vi "Get Tester Info.vi"(0 "TSM Context In":T1, 5 "Tester Type":string="RFPM", 11 "error in":errorcluster) -> (4 "TSM Context Out":T1, 6 "Resource Descriptors Exist?":bool, 8 "Resource Descriptors":string[](array[string]), 10 "Instrument Models":string[](array[string]), 15 "error out":errorcluster)   [LabVIEW 2023, in "RFCalAndFixtureCharact.Common.lvlib"]
uses:
  RFCalAndFixtureCharact.Common.lvlib
  <vilib>/NI_TestStand_SemiconductorModule/NI_TestStand_Semiconductor_Module.lvlibp/PinMap/General/SemiconductorModuleContext.ctl
  Global Data Id Prefix.vi
  <vilib>/NI_TestStand_SemiconductorModule/NI_TestStand_Semiconductor_Module.lvlibp
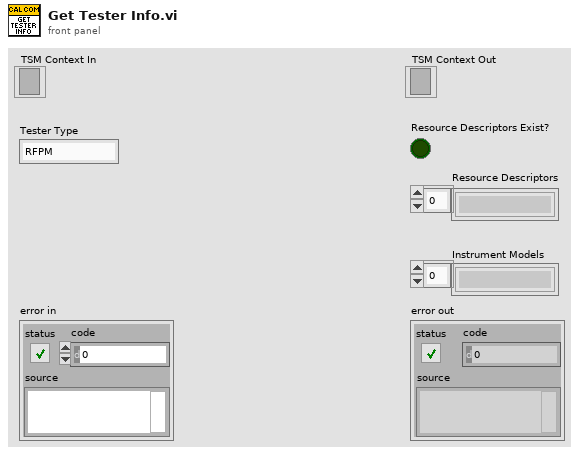
[diagram p1: front panel]
types:
  T1 = typedef "NI_TestStand_Semiconductor_Module.lvlibp/SemiconductorModuleContext.ctl" = refnum<k7>
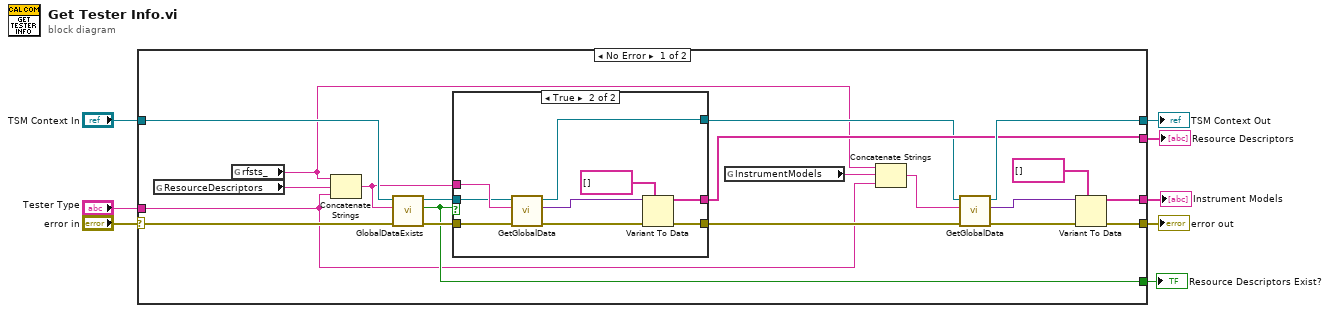
[diagram p0: block diagram]
diagram:
  n1 = case shown="No Error" "error in" {
    selector: "error in" -> [w21 w41]
    tunnel: [w28 w40] -> w8
    tunnel: [w27 _] -> w7
    tunnel: [w26 w41] -> w6
    tunnel: "TSM Context In" -> [w25 w40]
    tunnel: [w15 _] -> w4
    tunnel: [w22 _] -> w3
    tunnel: "Tester Type" -> [w13 _]
    frame No Error {
      n2 = global read "Global Data Id Prefix.vi" "ResourceDescriptors"() -> (w10:string)
      n3 = global read "Global Data Id Prefix.vi" "rfsts_"() -> (w9:string)
      n4 = Concatenate Strings(w9, w10, w13) -> (w14:string)
      n5 = call <vilib>:"GlobalDataExists.vi"("error in (no error)"=w21, "Data Id"=w14, "Semiconductor Module Context"=w25) -> ("error out"=w23:errorcluster, "Global Data Exists?"=w15:bool, "Semiconductor Module Context Out"=w24:T1)  [unwired: 6 in]
      n6 = case shown="True" w15 {
        tunnel: [_ w39] -> w27
        tunnel: w14 -> [_ w38]
        tunnel: w24 -> [w30 w37]
        tunnel: w23 -> [w29 w36]
        tunnel: [w30 w32] -> w20
        tunnel: [w29 w31] -> w19
        frame False {
        }
        frame True {
          n7 = call <vilib>:"GetGlobalData.vi"("error in (no error)"=w36, "Data Id"=w38, "Semiconductor Module Context"=w37) -> ("error out"=w35:errorcluster, "Data"=w34:variant, "Semiconductor Module Context Out"=w32:T1)  [unwired: 6 in]
          n8 = Variant To Data(error in=w35, type=string[] [], Variant=w34) -> (data=w39:string[], error out=w31:errorcluster)
        }
      }
      n9 = global read "Global Data Id Prefix.vi" "InstrumentModels"() -> (w12:string)
      n10 = Concatenate Strings(w9, w12, w13) -> (w11:string)
      n11 = call <vilib>:"GetGlobalData.vi"("error in (no error)"=w19, "Data Id"=w11, "Semiconductor Module Context"=w20) -> ("error out"=w17:errorcluster, "Data"=w16:variant, "Semiconductor Module Context Out"=w28:T1)  [unwired: 6 in]
      n12 = Variant To Data(error in=w17, type=string[] [], Variant=w16) -> (data=w22:string[], error out=w26:errorcluster)
    }
    frame Error {
    }
  }
  "TSM Context Out" <- w8
  "error out" <- w6
  "Resource Descriptors" <- w7
  "Resource Descriptors Exist?" <- w4
  "Instrument Models" <- w3
